vi "CW Transmit.vi"() -> ()   [LabVIEW 2024]
uses:
  <vilib>/Analysis/NI_AALBase.lvlib
panel:
  in  "Tab Control":enum32{"Control Tab"}(tab)
  out "mapped_values":variant=variant(" "=variant(string "        "), "A"=variant(string ". -   "), "B"=variant(string "- . . .   "), "C"=variant(string "- . - .   "), "D"=variant(string "- . .   "), "E"=variant(string ".   "), "F"=variant(string ". . - .   "), "G"=variant(string "- - .   "), "H"=variant(string ". . . .   "), "I"=variant(string ". .   "), "J"=variant(string ". - - -   "), "K"=variant(string "- . -   "), "L"=variant(string ". - . .   "), "M"=variant(string "- -   "), "N"=variant(string "- .   "), "O"=variant(string "- - -   "), "P"=variant(string ". - - .   "), "Q"=variant(string "- - . -   "), "R"=variant(string ". - .   "), "S"=variant(string ". . .   "), "T"=variant(string "-   "), "U"=variant(string ". . -   "), "V"=variant(string ". . . -   "), "W"=variant(string ". - -   "), "X"=variant(string "- . . -   "), "Y"=variant(string "- . - -   "), "Z"=variant(string "- - . .   "))
  out "Legenda":string="Parametru\t                              Valoare               \nDurata DOT (•)\t                                  0.1 s (100 ms)            \nDurata DASH (–)                                0.3 s (3 DOT)                      \nPauza simboluri\t                                 0.1 s                           \nPauza litere\t                                        0.3 s                          \nPauza cuvinte\t                                    0.7 s (7 DOTs)                    \nAmplitudine semnal\t                         0-5 V____                 "
  in  "Morse Code Message":string
  in  "Transmit":bool
  in  "stop":bool
  out "Signal Waveform":waveform(dbl)(graph)={"t0"=timestamp(0 s since 1904-01-01), "dt"=1e-05, "Y"=[]}
  out "Frequency (Hz)":i16(knob)=1000 scale=2.0..2000.0
  in  "Set Frequency":i16(knob)=1000 scale=51.0..2000.0
  in  "Set pulse length":i32(knob)=950 scale=100.0..10000.0
  out "Pulse length":i32(knob)=950 scale=100.0..10000.0
  in  "Set ampl.":dbl(knob)=5.0 scale=0.0..5.0
  out "Amplitude (V)":i16(knob)=5 scale=0.0..5.0
  in  "dt":dbl=100000.0 format="%#_13g"
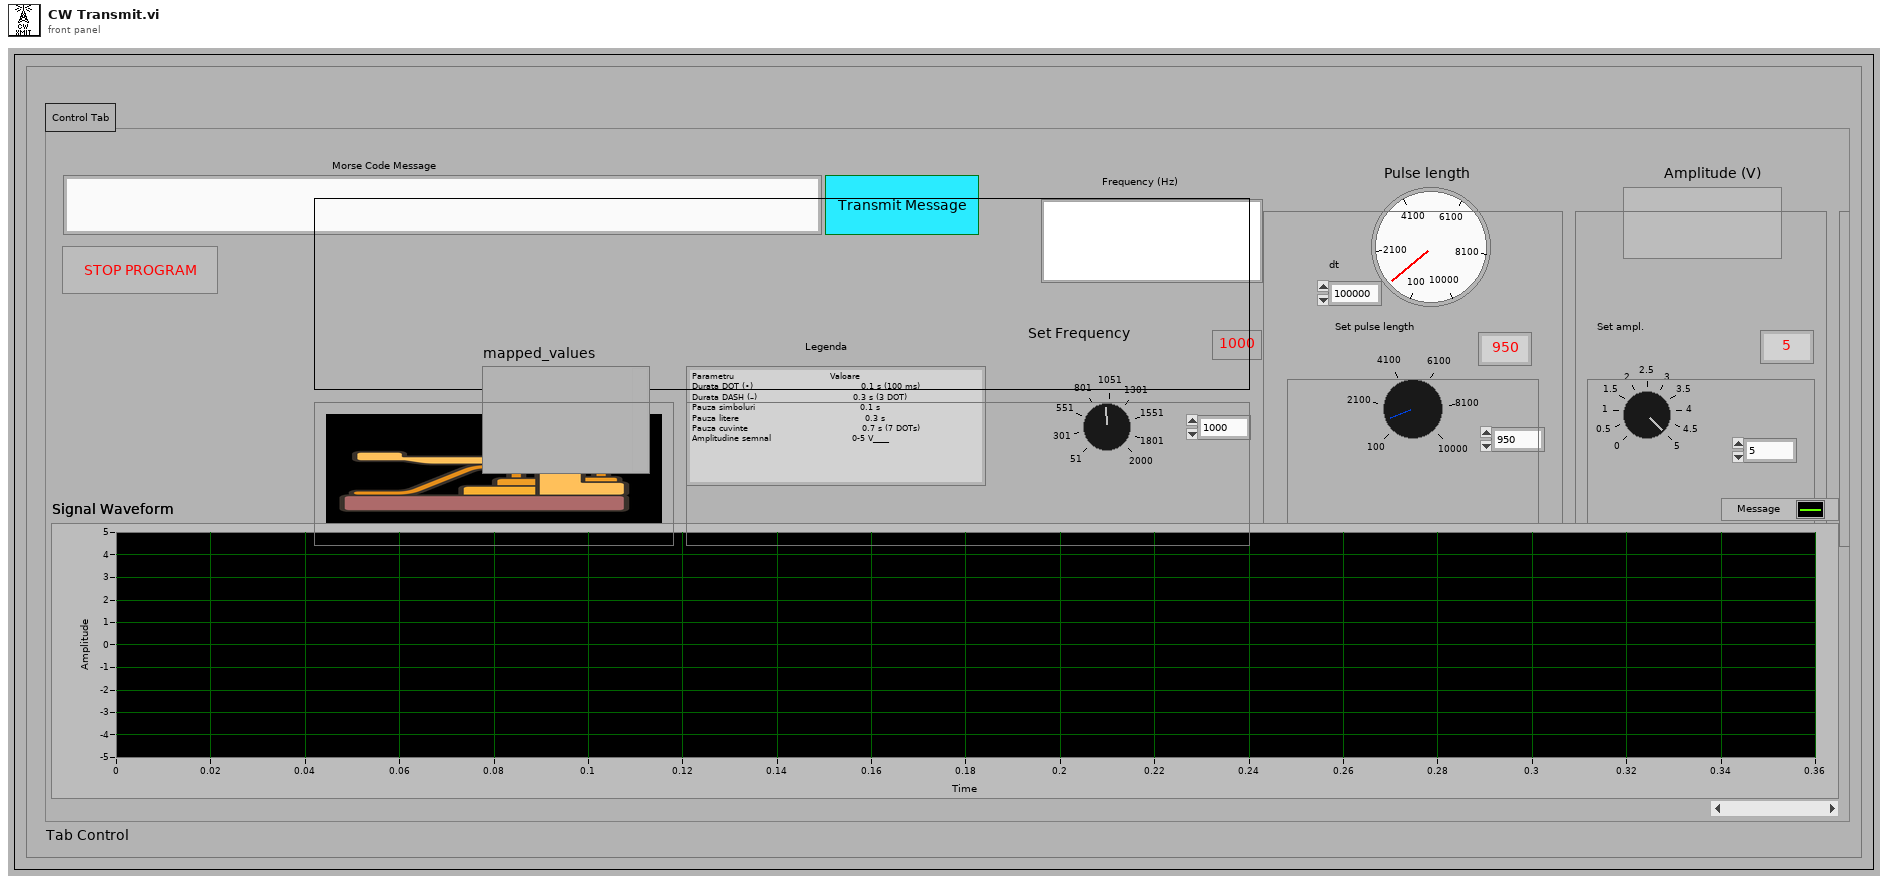
[diagram p1: front panel]
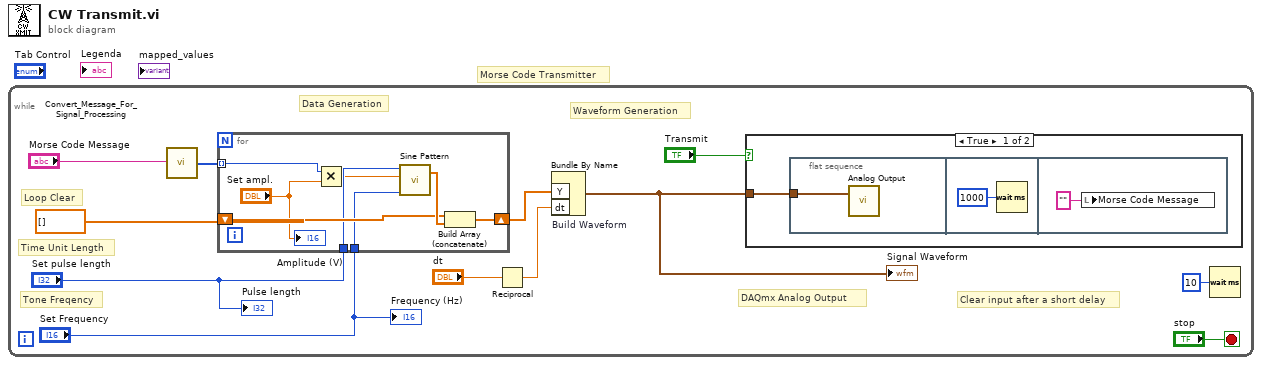
[diagram p0: block diagram]
diagram:
  # "Morse Code Transmitter"
  n1 = while {
    stop <- "stop" stop-if-true
    # "Clear input after a short delay"
    # "Waveform Generation"
    # "DAQmx Analog Output"
    # "Data Generation"
    # "Tone Freqency"
    # "Time Unit Length"
    # "Loop Clear"
    n2 = call "Convert_Message_For_Signal_Processing.vi"("String"="Morse Code Message") -> ("Array"=w3:i16[])
    n3 = for {
      shift-right: [w23] -> w5
      shift-left: dbl[] [] -> [w22]
      tunnel: w3 -> [w19] mode=indexing
      tunnel: "Set pulse length" -> [w21]
      tunnel: "Set Frequency" -> [w20]
      n4 = Multiply(x=w19, y="Set ampl.") -> (x*y=w18:dbl)
      n5 = call <vilib>:"Sine Pattern.vi"("cycles"=w20, "amplitude"=w18, "samples"=w21) -> ("Sinusoidal Pattern"=w24:dbl[])  [unwired: 1 in, 1 out]
      n6 = Build Array (concatenate)(w22, w24) -> (w23:dbl[])
      "Amplitude (V)" <- "Set ampl."
    }
    n7 = Reciprocal(x="dt") -> (1/x=w10:dbl)
    n8 = Bundle By Name "Build Waveform"("Y"=w5, "dt"=w10) -> (w2:waveform(dbl))  [unwired: 1 in]
    "Signal Waveform" <- w2
    n9 = case shown="True" "Transmit" {
      tunnel: w2 -> [w13 _]
      frame True {
        n10 = flat-sequence {
          tunnel: w13 -> [w14]
          frame #0 {
            n11 = call "Analog Output.vi"("output waveform"=w14) -> ()  [unwired: 2 in]
          }
          frame #1 {
            n12 = Wait (ms)(milliseconds to wait=u32 1000) -> ()  [unwired: 1 out]
          }
          frame #2 {
            n13 = local write "Morse Code Message"("" ("Morse Code Message")) -> ()
          }
        }
      }
      frame False {
      }
    }
    n14 = Wait (ms)(milliseconds to wait=u32 10) -> ()  [unwired: 1 out]
    "Frequency (Hz)" <- "Set Frequency"
    "Pulse length" <- "Set pulse length"
  }
